vi "TicTacToe_Checker.vi"(5 "BR":string, 6 "UL":string, 7 "MM":string, 8 "UM":string, 9 "MR":string, 10 "UR":string, 11 "BL":string, 12 "ML":string, 13 "BM":string) -> (17 "P1 or P2?":bool, 18 "\"GAME OVER\"":string)   [LabVIEW 2024]
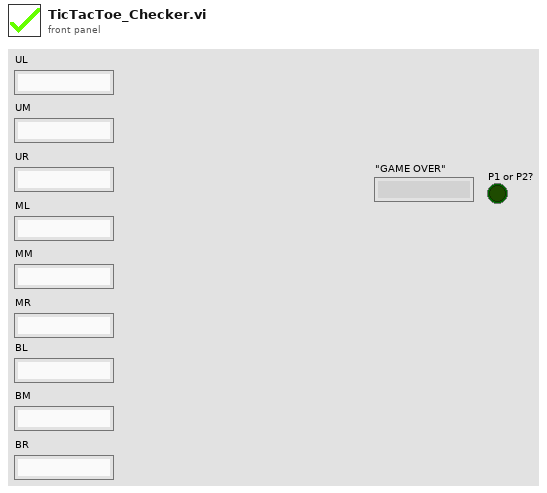
[diagram p1: front panel]
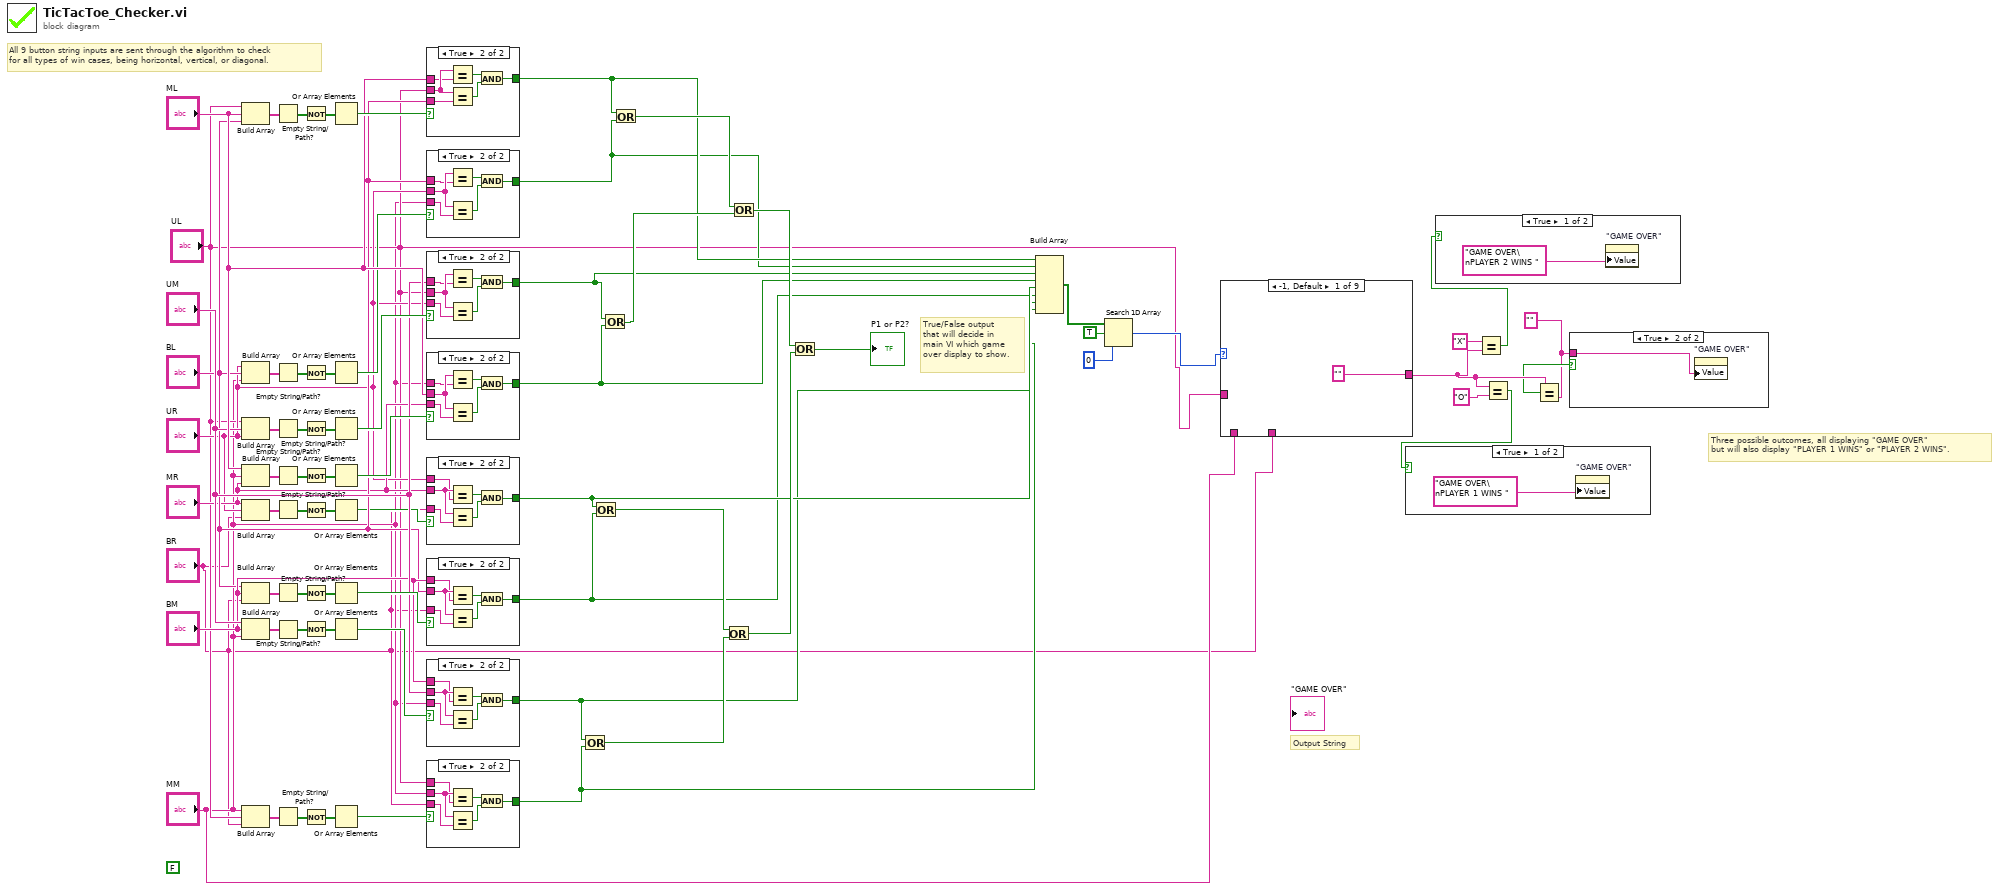
[diagram p0: block diagram]
diagram:
  w1 = "" ("y")
  (unwired) FALSE
  # "True/False output\nthat will decide in\nmain VI which game\nover display to show."
  # "All 9 button string inputs are sent through the algorithm to check\nfor all types of win cases, being horizontal, vertical, or diagonal."
  # "Output String"
  # "Three possible outcomes, all displaying \"GAME OVER\"\nbut will also display \"PLAYER 1 WINS\" or \"PLAYER 2 WINS\"."
  n1 = Build Array("UL", "ML", "BL") -> (w55:string[])
  n2 = Build Array("UR", "BL", "MM") -> (w40:string[])
  n3 = Build Array("UL", "UM", "UR") -> (w67:string[])
  n4 = Build Array("ML", "MM", "MR") -> (w63:string[])
  n5 = Build Array("MR", "UR", "BR") -> (w35:string[])
  n6 = Build Array("BL", "BM", "BR") -> (w59:string[])
  n7 = Build Array("UM", "BM", "MM") -> (w46:string[])
  n8 = Build Array("MM", "UL", "BR") -> (w50:string[])
  n9 = Empty String/Path?(string/path=w55) -> (empty?=w54:bool[])
  n10 = Empty String/Path?(string/path=w40) -> (empty?=w39:bool[])
  n11 = Empty String/Path?(string/path=w67) -> (empty?=w66:bool[])
  n12 = Empty String/Path?(string/path=w63) -> (empty?=w62:bool[])
  n13 = Empty String/Path?(string/path=w35) -> (empty?=w34:bool[])
  n14 = Empty String/Path?(string/path=w59) -> (empty?=w58:bool[])
  n15 = Empty String/Path?(string/path=w46) -> (empty?=w45:bool[])
  n16 = Empty String/Path?(string/path=w50) -> (empty?=w49:bool[])
  n17 = Not(x=w54) -> (.not. x?=w53:bool[])
  n18 = Not(x=w39) -> (.not. x?=w38:bool[])
  n19 = Not(x=w66) -> (.not. x?=w65:bool[])
  n20 = Not(x=w62) -> (.not. x?=w61:bool[])
  n21 = Not(x=w34) -> (.not. x?=w33:bool[])
  n22 = Not(x=w58) -> (.not. x?=w57:bool[])
  n23 = Not(x=w45) -> (.not. x?=w44:bool[])
  n24 = Not(x=w49) -> (.not. x?=w48:bool[])
  n25 = Or Array Elements(Boolean array=w53) -> (logical OR=w52:bool)
  n26 = Or Array Elements(Boolean array=w38) -> (logical OR=w37:bool)
  n27 = Or Array Elements(Boolean array=w65) -> (logical OR=w64:bool)
  n28 = Or Array Elements(Boolean array=w61) -> (logical OR=w60:bool)
  n29 = Or Array Elements(Boolean array=w33) -> (logical OR=w32:bool)
  n30 = Or Array Elements(Boolean array=w57) -> (logical OR=w56:bool)
  n31 = Or Array Elements(Boolean array=w44) -> (logical OR=w43:bool)
  n32 = Or Array Elements(Boolean array=w48) -> (logical OR=w47:bool)
  n33 = case shown="True" w52 {
    tunnel: "UL" -> [_ w73]
    tunnel: "ML" -> [_ w72]
    tunnel: "BL" -> [_ w71]
    tunnel: [_ w68] -> w22
    frame False {
    }
    frame True {
      n34 = Equal?(x=w73, y=w72) -> (x = y?=w70:bool)
      n35 = Equal?(x=w73, y=w71) -> (x = y?=w69:bool)
      n36 = And(x=w70, y=w69) -> (x .and. y?=w68:bool)
    }
  }
  n37 = case shown="True" w37 {
    tunnel: "UR" -> [_ w79]
    tunnel: "BL" -> [_ w78]
    tunnel: "MM" -> [_ w77]
    tunnel: [_ w74] -> w21
    frame False {
    }
    frame True {
      n38 = Equal?(x=w79, y=w78) -> (x = y?=w76:bool)
      n39 = Equal?(x=w79, y=w77) -> (x = y?=w75:bool)
      n40 = And(x=w76, y=w75) -> (x .and. y?=w74:bool)
    }
  }
  n41 = case shown="True" w64 {
    tunnel: "UL" -> [_ w85]
    tunnel: "UM" -> [_ w84]
    tunnel: "UR" -> [_ w83]
    tunnel: [_ w80] -> w20
    frame False {
    }
    frame True {
      n42 = Equal?(x=w85, y=w84) -> (x = y?=w82:bool)
      n43 = Equal?(x=w85, y=w83) -> (x = y?=w81:bool)
      n44 = And(x=w82, y=w81) -> (x .and. y?=w80:bool)
    }
  }
  n45 = case shown="True" w60 {
    tunnel: "ML" -> [_ w91]
    tunnel: "MM" -> [_ w90]
    tunnel: "MR" -> [_ w89]
    tunnel: [_ w86] -> w19
    frame False {
    }
    frame True {
      n46 = Equal?(x=w91, y=w90) -> (x = y?=w88:bool)
      n47 = Equal?(x=w91, y=w89) -> (x = y?=w87:bool)
      n48 = And(x=w88, y=w87) -> (x .and. y?=w86:bool)
    }
  }
  n49 = case shown="True" w32 {
    tunnel: "MR" -> [_ w97]
    tunnel: "UR" -> [_ w96]
    tunnel: "BR" -> [_ w95]
    tunnel: [_ w92] -> w18
    frame False {
    }
    frame True {
      n50 = Equal?(x=w97, y=w96) -> (x = y?=w94:bool)
      n51 = Equal?(x=w97, y=w95) -> (x = y?=w93:bool)
      n52 = And(x=w94, y=w93) -> (x .and. y?=w92:bool)
    }
  }
  n53 = case shown="True" w56 {
    tunnel: "BL" -> [_ w103]
    tunnel: "BM" -> [_ w102]
    tunnel: "BR" -> [_ w101]
    tunnel: [_ w98] -> w17
    frame False {
    }
    frame True {
      n54 = Equal?(x=w103, y=w102) -> (x = y?=w100:bool)
      n55 = Equal?(x=w103, y=w101) -> (x = y?=w99:bool)
      n56 = And(x=w100, y=w99) -> (x .and. y?=w98:bool)
    }
  }
  n57 = case shown="True" w43 {
    tunnel: "UM" -> [_ w109]
    tunnel: "BM" -> [_ w108]
    tunnel: "MM" -> [_ w107]
    tunnel: [_ w104] -> w16
    frame False {
    }
    frame True {
      n58 = Equal?(x=w109, y=w108) -> (x = y?=w106:bool)
      n59 = Equal?(x=w109, y=w107) -> (x = y?=w105:bool)
      n60 = And(x=w106, y=w105) -> (x .and. y?=w104:bool)
    }
  }
  n61 = case shown="True" w47 {
    tunnel: "MM" -> [_ w115]
    tunnel: "UL" -> [_ w114]
    tunnel: "BR" -> [_ w113]
    tunnel: [_ w110] -> w15
    frame False {
    }
    frame True {
      n62 = Equal?(x=w115, y=w114) -> (x = y?=w112:bool)
      n63 = Equal?(x=w115, y=w113) -> (x = y?=w111:bool)
      n64 = And(x=w112, y=w111) -> (x .and. y?=w110:bool)
    }
  }
  n65 = Or(x=w16, y=w15) -> (x .or. y?=w26:bool)
  n66 = Or(x=w18, y=w17) -> (x .or. y?=w27:bool)
  n67 = Or(x=w20, y=w19) -> (x .or. y?=w28:bool)
  n68 = Or(x=w22, y=w21) -> (x .or. y?=w29:bool)
  n69 = Or(x=w27, y=w26) -> (x .or. y?=w24:bool)
  n70 = Or(x=w29, y=w28) -> (x .or. y?=w25:bool)
  n71 = Or(x=w25, y=w24) -> (x .or. y?=→"P1 or P2?":bool)
  n72 = Build Array(w22, w21, w20, w19, w18, w17, w16, w15) -> (w14:bool[])
  n73 = Search 1D Array(1D array=w14, element=TRUE, start index (0)=0) -> (index of element=w11:i32)
  n74 = case shown="-1, Default" w11 {
    tunnel: "UL" -> [_ w117 _ w119 _ _ _ _ w124]
    tunnel: "MM" -> [_ _ w118 _ w120 _ _ w123 _]
    tunnel: "BR" -> [_ _ _ _ _ w121 w122 _ _]
    tunnel: ["" w117 w118 w119 w120 w121 w122 w123 w124] -> w3
    frame -1, Default {
    }
    frame 0 {
    }
    frame 1 {
    }
    frame 2 {
    }
    frame 3 {
    }
    frame 4 {
    }
    frame 5 {
    }
    frame 6 {
    }
    frame 7 {
    }
  }
  n75 = Equal?(x="X", y=w3) -> (x = y?=w5:bool)
  n76 = case shown="True" w5 {
    frame True {
      n77 = property on="\"GAME OVER\"" class="Str"("Value"="GAME OVER\nPLAYER 2 WINS ") -> ()  [unwired: 2 in, 2 out]
    }
    frame False {
    }
  }
  n78 = Equal?(x=w3, y="O") -> (x = y?=w4:bool)
  n79 = case shown="True" w4 {
    frame True {
      n80 = property on="\"GAME OVER\"" class="Str"("Value"="GAME OVER\nPLAYER 1 WINS ") -> ()  [unwired: 2 in, 2 out]
    }
    frame False {
    }
  }
  n81 = Equal?(x=w3, y=w1) -> (x = y?=w2:bool)
  n82 = case shown="True" w2 {
    tunnel: w1 -> [_ w127]
    frame False {
    }
    frame True {
      n83 = property on="\"GAME OVER\"" class="Str"("Value"=w127) -> ()  [unwired: 2 in, 2 out]
    }
  }
